vi "search2Darray_noReps.vi"(9 "target":dbl, 11 "Array":dbl[][](array[numeric])) -> (2 "indices":i32[][](array[numeric]))   [LabVIEW 2017]
panel:
  # "Can't find repeating elements!!!!!!!!!!!!!!!!!!!!!!!!!!"
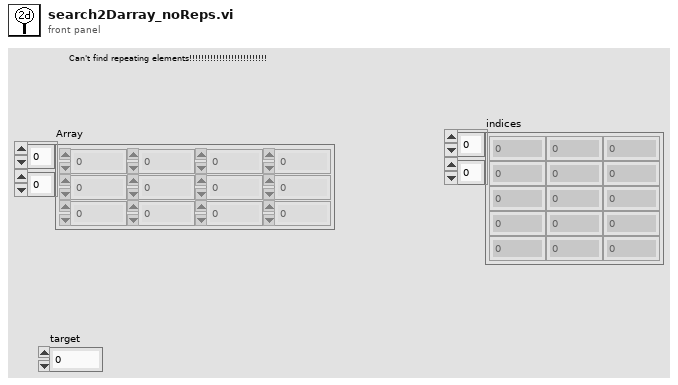
[diagram p1: front panel]
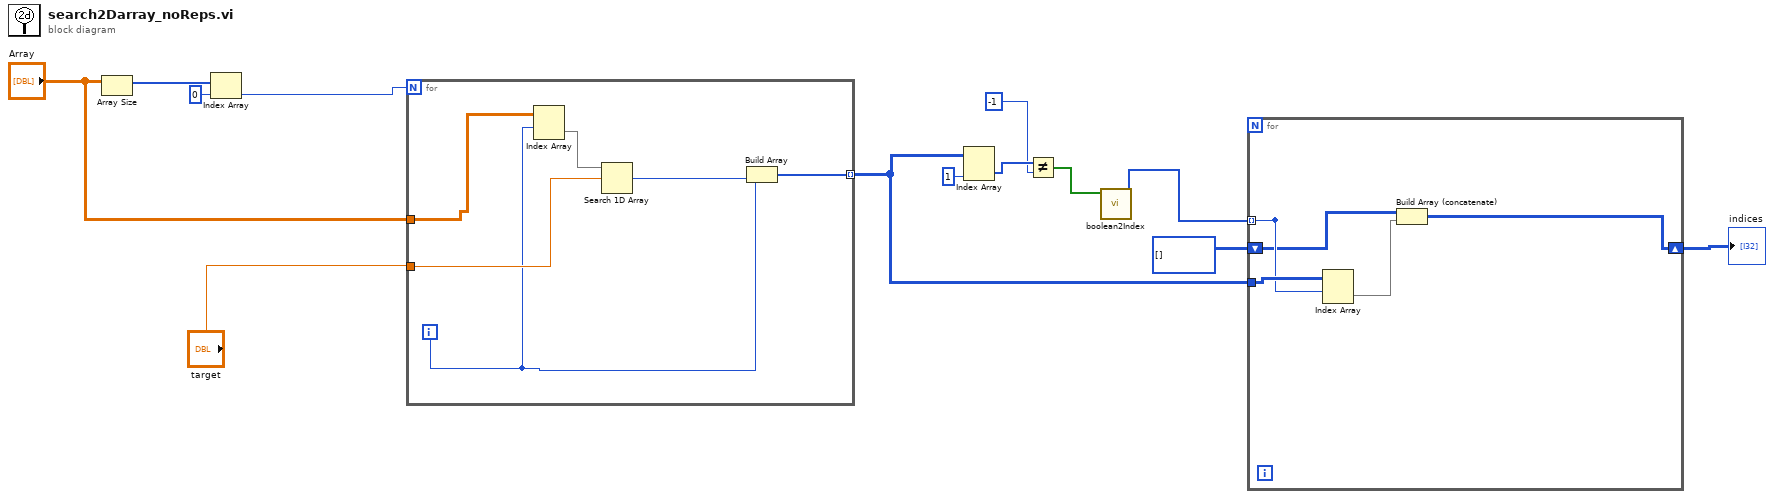
[diagram p0: block diagram]
diagram:
  n1 = Array Size(array="Array") -> (size(s)=w13:i32[])
  n2 = Index Array(array=w13, index=0) -> (element=w11:i32)
  n3 = for {
    N: w11 -> [_]
    tunnel: "Array" -> [w19]
    tunnel: "target" -> [w17]
    tunnel: [w14] -> w3 mode=indexing
    i -> [w15]
    n4 = Index Array(array=w19, index (row)=w15) -> (element=w18:dbl[])  [unwired: 1 in]
    n5 = Search 1D Array(1D array=w18, element=w17) -> (index of element=w16:i32)  [unwired: 1 in]
    n6 = Build Array(w15, w16) -> (w14:i32[])
  }
  n7 = Index Array(array=w3, index (col)=1 ("disabled index (col)")) -> (element=w7:i32[])  [unwired: 1 in]
  n8 = Not Equal?(x=w7, y=-1) -> (x != y?=w5:bool[])
  n9 = call "boolean2Index.vi"("boolean"=w5) -> ("index"=w4:i32[])  [unwired: 10 in]
  n10 = for {
    tunnel: [w23] -> _ mode=indexing
    tunnel: w4 -> [w23] mode=indexing
    tunnel: w3 -> [w24]
    shift-right: [w20] -> w1
    shift-left: i32[][] [] ("element") -> [w21]
    n11 = Index Array(array=w24, index (row)=w23) -> (element=w22:i32[])  [unwired: 1 in]
    n12 = Build Array (concatenate)(w21, w22) -> (w20:i32[][])
  }
  "indices" <- w1
